vi "Wrapper_Destroy.vi"(0 "Wrapper":u32) -> ()   [LabVIEW 2017]
uses:
  OmniDriver32.dll
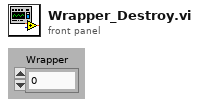
[diagram p1: front panel]
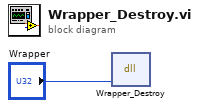
[diagram p0: block diagram]
diagram:
  n1 = dll-call lib="OmniDriver32.dll" fn="Wrapper_Destroy" label="Wrapper.Destroy"("Wrapper"="Wrapper") -> ()  [unwired: 4 in, 3 out]
